vi "iRobot Navigation Target (Filtered).vi"() -> ()   [LabVIEW 2013]
uses:
  iRobot Sensors.ctl
  iRobot/Sensor/Charging State.ctl
  Accel Filtered.ctl
  iRobot Navigation State Machine.lvsc/StatechartState.ctl
  iRobot Navigation State Machine.lvsc/State.ctl
  iRobot Navigation State Machine.lvsc/Inputs.ctl
  Accelerometer.ctl
  iRobot/Sensor/Sensor Group 6.ctl
  iRobot/Sensor/Bumps + Wheel Drops.ctl
  iRobot/Sensor/Low-Side Driver + Wheel Overcurrent.ctl
  iRobot/Sensor/Buttons.ctl
  iRobot/Sensor/Cargo Bay Digital Inputs.ctl
  iRobot/Sensor/Charging Sources Available.ctl
  iRobot/Sensor/OI Mode.ctl
  <vilib>/Statechart/Common/IntGuid.ctl
  <vilib>/Statechart/Common/DbgID.ctl
  <vilib>/myRIO/Common/Instrument Driver Framework/myRIO v1.0/UART/vis/myRIO v1.0 Close UART.vi
  <vilib>/myRIO/Common/Instrument Driver Framework/myRIO v1.0/myRIO v1.1 Open.vi
  iRobot Navigation State Machine.lvsc/CompanionDiagram.vi
  iRobot Navigation State Machine.lvsc/CompanionDiagram.vi/38/SC Main.vi
  <vilib>/myRIO/Common/Instrument Driver Framework/Utilities/vis/FPGA Ref Manager.vi
  <vilib>/myRIO/Common/Instrument Driver Framework/myRIO v1.0/myRIO v1.0 Reset FPGA.vi
  iRobot Navigation State Machine.lvsc/Trigger.ctl
  <vilib>/Statechart/Infrastructure/RTStatechart/RunTime SCN.xnode
  iRobot Navigation State Machine.lvsc/Outputs.ctl
  iRobot Navigation State Machine.lvsc
  <vilib>/myRIO/Instrument Drivers/Utilities/Utilities.lvlib
  <vilib>/Statechart/Common/NI_SC_LVSCCommonFiles.lvlib
panel:
  in  "Reset Peak Deg":bool
  out "Horiz. Peak Angle 2":dbl
  in  "Delta Mag. Thresh. 2":dbl
  in  "Deg. Accel. Thresh.":dbl
  out "Horiz. Peak Angle":dbl
  in  "Reset Accel Max":bool
  in  "Reset Delta Max":bool
  in  "Tab Control":T1(tab)
  out "iRobot Sensors (graphical)":T2 {"Filtered Delta Max"."All Mag" format="%_3f"; "Filtered Delta Max"."Vert Mag" format="%_3f"; "Filtered Delta Max"."x axis (g)" format="%_3f"; "Filtered Delta Max"."y axis (g)" format="%_3f"; "Filtered Delta Max"."z axis (g)" format="%_3f"; "Filtered Delta Max"."Horiz Mag" format="%_3f"; "Filtered Accel Max"."All Mag" format="%_3f"; "Filtered Accel Max"."Vert Mag" format="%_3f"; "Filtered Accel Max"."x axis (g)" format="%_3f"; "Filtered Accel Max"."y axis (g)" format="%_3f"; "Filtered Accel Max"."z axis (g)" format="%_3f"; "Filtered Accel Max"."Horiz Mag" format="%_3f"; "Right Wheel (mm/s)" scale=-500.0..500.0; "Left Wheel (mm/s)" scale=-500.0..500.0}
  in  "Full Mode":bool
  out "Active States":T6
  out "error out":errorcluster
  in  "Wheel Speed (mm/s)":i16(slide)=100 scale=0.0..500.0
  in  "accel smoothing (0-1)":dbl=1.0
  in  "accel HPF (0-1)":dbl=0.7
  in  "stop":bool
  out "Target Running":bool
  # "Battery"
  # "Set to 1 to disable"
  # "Set to 0 to disable ???"
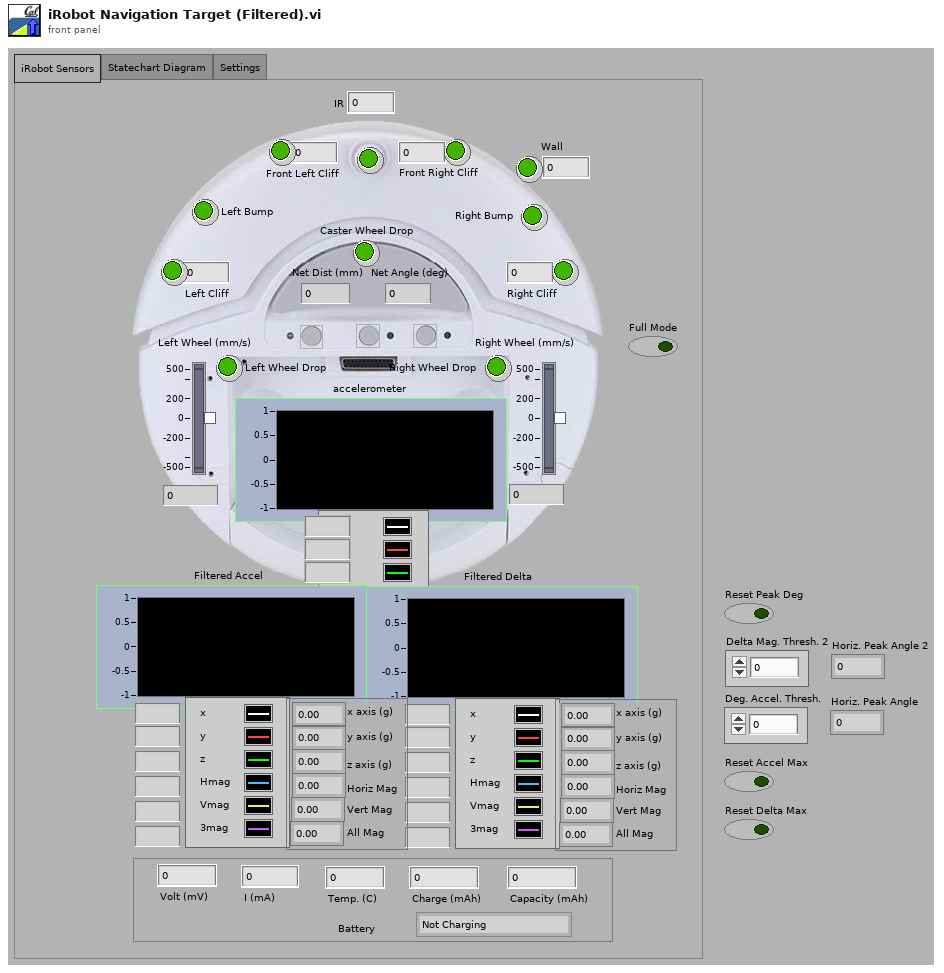
[diagram p1: front panel]
types:
  T1 = enum32{"iRobot Sensors", "Statechart Diagram", "Settings"}
  T2 = typedef "iRobot Sensors.ctl" = cluster{"Caster Wheel Drop":bool, "Left Wheel Drop":bool, "Right Wheel Drop":bool, "Left Bump":bool, "Right Bump":bool, "Left Cliff":bool, "Front Left Cliff":bool, "Front Right Cliff":bool, "Right Cliff":bool, "Wall":bool, "Net Dist (mm)":i32, "Net Angle (deg)":i32, "Wall":u16, "Left Cliff":u16, "Front Left Cliff":u16, "Front Right Cliff":u16, "Right Cliff":u16, "Left Wheel (mm/s)":i16, "Right Wheel (mm/s)":i16, "accelerometer":T3, "Virtual Wall":bool, "Volt (mV)":u16, "I (mA)":i16, "Temp. (C)":i8, "Charge (mAh)":u16, "Capacity (mAh)":u16, "Charging State":T4, "IR":u8, "Filtered Accel":cluster{"x axis (g)":dbl, "y axis (g)":dbl, "z axis (g)":dbl, "Horiz Mag":dbl, "Vert Mag":dbl, "All Mag":dbl}, "Filtered Delta":cluster{"x axis (g)":dbl, "y axis (g)":dbl, "z axis (g)":dbl, "Horiz Mag":dbl, "Vert Mag":dbl, "All Mag":dbl}, "Filtered Accel Max":T5, "Filtered Delta Max":T5}
  T3 = typedef "Accelerometer.ctl" = cluster{"x axis (g)":dbl, "y axis (g)":dbl, "z axis (g)":dbl}
  T4 = typedef "Charging State.ctl" = enum16{"Not Charging", "Reconditioning Charging", "Full Charging", "Trickle Charging", "Waiting", "Charging Fault Condition"}
  T5 = typedef "Accel Filtered.ctl" = cluster{"x axis (g)":dbl, "y axis (g)":dbl, "z axis (g)":dbl, "Horiz Mag":dbl, "Vert Mag":dbl, "All Mag":dbl}
  T6 = typedef "iRobot Navigation State Machine.lvsc/StatechartState.ctl" = T7[]
  T7 = typedef "iRobot Navigation State Machine.lvsc/State.ctl" = enum16{"NI.SC.Initial", "NI.SC.History", "NI.SC.ShallowHistory", "NI.SC.Terminal", "Pause", "Run", "Pause\\Detect Play Button\\Pause;\nWait for\nbutton\nrelease", "Pause\\Detect Play Button\\Unpause;\nwait for\nbutton release", "Pause\\Detect Play Button\\Unpause;\nwait for\nbutton press", "Run\\Detect Obstacles\\Return Right", "Run\\Detect Obstacles\\Return Left", "Run\\Detect Obstacles\\Move Forward", "Run\\Detect Obstacles\\Turn Right", "Run\\Detect Obstacles\\Turn Left", "Run\\Detect Obstacles\\Backup", "Run\\Detect Obstacles\\Drive"}
  T8 = typedef "iRobot UART Port Type.ctl" = refnum<visa-resource-name>
  T9 = typedef "NI_SC_LVSCCommonFiles.lvlib/IntGuid.ctl" = cluster{"Data1":u32, "Data2":u16, "Data3":u16, "Data4":u8, "Data5":u8, "Data6":u8, "Data11":u8, "Data9":u8, "Data10":u8, "Data8":u8, "Data7":u8}
  T10 = typedef "NI_SC_LVSCCommonFiles.lvlib/DbgID.ctl" = cluster{"VIRef":u32, "IntGUID":T9}
  T11 = typedef "iRobot Navigation State Machine.lvsc/Inputs.ctl" = cluster{"net distance (mm)":i32, "net angle (deg)":i32, "Max Wheel Speed (mm/s)":i16, "accelerometer":T3, "iRobot Sensors":T12, "Is Simulator?":bool, "Filtered Accelerometer":T5, "Filtered Accel Delta":T5}
  T12 = typedef "Sensor Group 6.ctl" = cluster{"Bumps + Wheel Drops":T13, "Wall":bool, "Cliff Left":bool, "Cliff Front Left":bool, "Cliff Front Right":bool, "Cliff Right":bool, "Virtual Wall":bool, "Low-Side Driver + Wheel Overcurrent":T14, "Infrared":u8, "Buttons":T15, "Distance (mm)":i32, "Angle (deg)":i32, "Charging State":T4, "Voltage (mV)":u16, "Current (mA)":i16, "Battery Temperature (deg C)":i8, "Battery Charge (mAh)":u16, "Battery Capacity (mAh)":u16, "Wall Signal (0-4095)":u16, "Cliff Left Signal (0-4095)":u16, "Cliff Front Left Signal (0-4095)":u16, "Cliff Front Right Signal (0-4095)":u16, "Cliff Right Signal (0-4095)":u16, "Cargo Bay Digital Inputs":T16, "Cargo Bay Analog Signal (0-1023)":u16, "Charging Sources Available":T17, "OI Mode":T18, "Song Number":u8, "Song Playing":bool, "Number of Stream Packets":u8, "Requested Velocity (mm/s)":i16, "Requested Radius (mm)":i16, "Requested Right Wheel Velocity (mm/s)":i16, "Requested Left Wheel Velocity (mm/s)":i16}
  T13 = typedef "Bumps + Wheel Drops.ctl" = cluster{"Wheeldrop Caster":bool, "Wheeldrop Left":bool, "Wheeldrop Right":bool, "Bump Left":bool, "Bump Right":bool}
  T14 = typedef "Low-Side Driver + Wheel Overcurrent.ctl" = cluster{"Low-Side Driver 0":bool, "Low-Side Driver 1":bool, "Low-Side Driver 2":bool, "Left Wheel":bool, "Right Wheel":bool}
  T15 = typedef "Buttons.ctl" = cluster{"Advance":bool, "Play":bool}
  T16 = typedef "Cargo Bay Digital Inputs.ctl" = cluster{"Digital Input 0":bool, "Digital Input 1":bool, "Digital Input 2":bool, "Digital Input 3":bool, "Device Detect":bool}
  T17 = typedef "Charging Sources Available.ctl" = cluster{"Internal Charger":bool, "Home Base":bool}
  T18 = typedef "OI Mode.ctl" = enum16{"Off", "Passive", "Safe", "Full"}
  T19 = typedef "iRobot Navigation State Machine.lvsc/Outputs.ctl" = cluster{"Left Wheel Speed (mm/s)":i16, "Right Wheel Speed (mm/s)":i16}
  T20 = cluster{"[0]":dbl, "[1]":dbl, "[2]":dbl, "[3]":dbl, "[4]":dbl, "[5]":dbl}
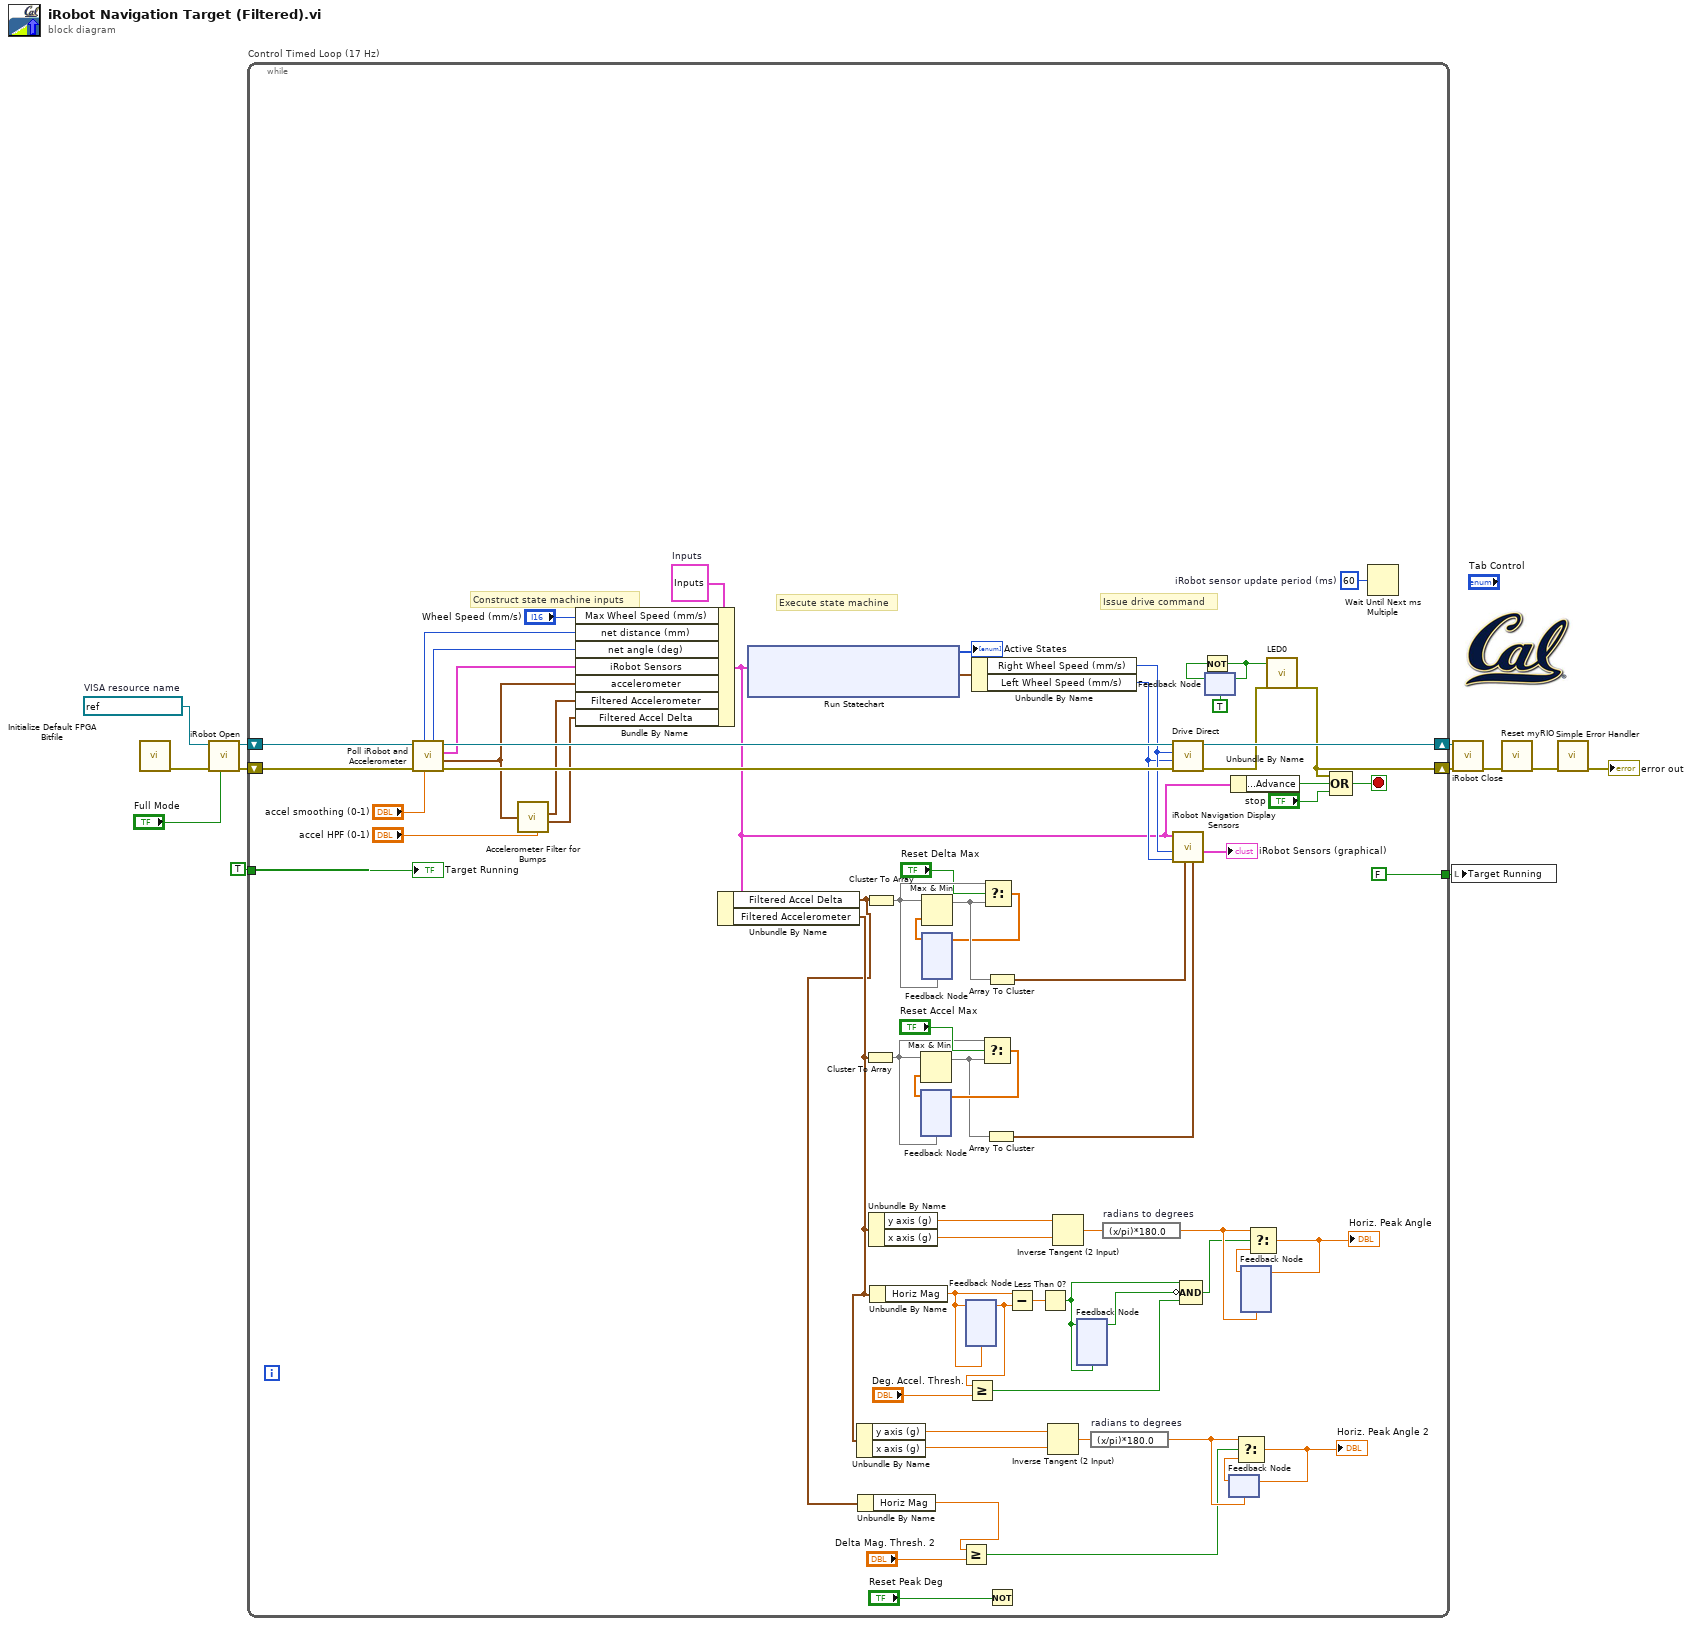
[diagram p0: block diagram]
diagram:
  w6 = refnum<visa-resource-name> "ASRL1::INSTR"  # VISA resource name
  n1 = call <vilib>:"Initialize Default FPGA Bitfile.vi"() -> ("error out"=w4:errorcluster)  [unwired: 11 in]
  n2 = call "iRobot Open.vi"("Full Mode"="Full Mode", "error in (no error)"=w4, "UART port in"=w6) -> ("error out"=w11:errorcluster, "UART port out"=w10:T8)  [unwired: 7 in]
  n3 = while "Control Timed Loop (17 Hz)" {
    shift-right: [w82] -> w12
    shift-left: w10 -> [w77]
    shift-right: [w64] -> w7
    shift-left: w11 -> [w76]
    tunnel: TRUE ("stop") -> [w70]
    tunnel: [FALSE ("stop")] -> w8
    stop <- w81 stop-if-true
    w57 = u32 60  # iRobot sensor update period (ms)
    w79 = T11 {"net distance (mm)"=0, "net angle (deg)"=0, "Max Wheel Speed (mm/s)"=0, "accelerometer"={"x axis (g)"=0.0, "y axis (g)"=0.0, "z axis (g)"=0.0}, "iRobot Sensors"={"Bumps + Wheel Drops"={"Wheeldrop Caster"=FALSE, "Wheeldrop Left"=FALSE, "Wheeldrop Right"=FALSE, "Bump Left"=FALSE, "Bump Right"=FALSE}, "Wall"=FALSE, "Cliff Left"=FALSE, "Cliff Front Left"=FALSE, "Cliff Front Right"=FALSE, "Cliff Right"=FALSE, "Virtual Wall"=FALSE, "Low-Side Driver + Wheel Overcurrent"={"Low-Side Driver 0"=FALSE, "Low-Side Driver 1"=FALSE, "Low-Side Driver 2"=FALSE, "Left Wheel"=FALSE, "Right Wheel"=FALSE}, "Infrared"=0, "Buttons"={"Advance"=FALSE, "Play"=FALSE}, "Distance (mm)"=0, "Angle (deg)"=0, "Charging State"=enum."Not Charging", "Voltage (mV)"=0, "Current (mA)"=0, "Battery Temperature (deg C)"=0, "Battery Charge (mAh)"=0, "Battery Capacity (mAh)"=0, "Wall Signal (0-4095)"=0, "Cliff Left Signal (0-4095)"=0, "Cliff Front Left Signal (0-4095)"=0, "Cliff Front Right Signal (0-4095)"=0, "Cliff Right Signal (0-4095)"=0, "Cargo Bay Digital Inputs"={"Digital Input 0"=FALSE, "Digital Input 1"=FALSE, "Digital Input 2"=FALSE, "Digital Input 3"=FALSE, "Device Detect"=FALSE}, "Cargo Bay Analog Signal (0-1023)"=0, "Charging Sources Available"={"Internal Charger"=FALSE, "Home Base"=FALSE}, "OI Mode"=enum."Off", "Song Number"=0, "Song Playing"=FALSE, "Number of Stream Packets"=0, "Requested Velocity (mm/s)"=0, "Requested Radius (mm)"=0, "Requested Right Wheel Velocity (mm/s)"=0, "Requested Left Wheel Velocity (mm/s)"=0}, "Is Simulator?"=FALSE, "Filtered Accelerometer"={"x axis (g)"=0.0, "y axis (g)"=0.0, "z axis (g)"=0.0, "Horiz Mag"=0.0, "Vert Mag"=0.0, "All Mag"=0.0}, "Filtered Accel Delta"={"x axis (g)"=0.0, "y axis (g)"=0.0, "z axis (g)"=0.0, "Horiz Mag"=0.0, "Vert Mag"=0.0, "All Mag"=0.0}}  # Inputs
    # "Issue drive command"
    # "Execute state machine"
    # "Construct state machine inputs"
    n4 = call "Poll iRobot and Accelerometer.vi"("accel smoothing (0-1)"="accel smoothing (0-1)", "error in"=w76, "UART port in"=w77) -> ("error out"=w75:errorcluster, "Acceleration (g)"=w54:T3, "iRobot SensorGroup6"=w63:T12, "UART port out"=w74:T8, "net angle (deg)"=w72:i32, "net distance (mm)"=w73:i32)  [unwired: 3 in]
    n5 = call "Accelerometer Filter for Bumps.vi"("filter factor (0-1)"="accel HPF (0-1)", "accelerometer (g)"=w54) -> ("filtered out"=w53:T5, "abs delta"=w52:T5)  [unwired: 4 in]
    n6 = Bundle By Name(cluster=w79, "Max Wheel Speed (mm/s)"="Wheel Speed (mm/s)", "net distance (mm)"=w73, "net angle (deg)"=w72, "iRobot Sensors"=w63, "accelerometer"=w54, "Filtered Accelerometer"=w53, "Filtered Accel Delta"=w52) -> (w47:T11)
    n7 = Unbundle By Name(w47) -> ("Filtered Accel Delta"=w22:T5, "Filtered Accelerometer"=w23:T5)
    n8 = xnode "Run Statechart"("Inputs"=w47) -> ("Outputs"=w80:T19, "Active States"=→"Active States":T6)  [unwired: 2 in, 1 out]
    n9 = Unbundle By Name(w23) -> ("y axis (g)"=w20:dbl, "x axis (g)"=w19:dbl)
    n10 = Unbundle By Name(w22) -> ("Horiz Mag"=w21:dbl)
    n11 = Cluster To Array(cluster=w23) -> (array=w42:dbl[])
    n12 = Cluster To Array(cluster=w22) -> (array=w49:dbl[])
    n13 = Unbundle By Name(w23) -> ("y axis (g)"=w16:dbl, "x axis (g)"=w15:dbl)
    n14 = Unbundle By Name(w23) -> ("Horiz Mag"=w30:dbl)
    n15 = feedback #1(w42) -> (w43:dbl[])
    n16 = Max & Min(x=w42, y=w43) -> (max(x,y)=w40:dbl[])  [unwired: 1 out]
    n17 = feedback #2(w49) -> (w48:dbl[])
    n18 = Max & Min(x=w49, y=w48) -> (max(x,y)=w51:dbl[])  [unwired: 1 out]
    n19 = Greater Or Equal?(x=w21, y="Delta Mag. Thresh. 2") -> (x >= y?=w13:bool)
    n20 = feedback #3(w30) -> (w28:dbl)
    n21 = feedback-in #3(w30) -> ()
    n22 = Greater Or Equal?(x=w28, y="Deg. Accel. Thresh.") -> (x >= y?=w31:bool)
    n23 = Unbundle By Name(w80) -> ("Right Wheel Speed (mm/s)"=w61:i16, "Left Wheel Speed (mm/s)"=w60:i16)
    n24 = Select(t=w42, s="Reset Accel Max", f=w40) -> (s? t:f=w41:dbl[])
    n25 = feedback-in #1(w41) -> ()
    n26 = Select(t=w49, s="Reset Delta Max", f=w51) -> (s? t:f=w50:dbl[])
    n27 = feedback-in #2(w50) -> ()
    n28 = Array To Cluster(array=w40) -> (cluster=w39:T20)
    n29 = Array To Cluster(array=w51) -> (cluster=w46:T20)
    n30 = Not(x="Reset Peak Deg") -> ()  [unwired: 1 out]
    n31 = Subtract(x=w30, y=w28) -> (x-y=w35:dbl)
    n32 = Less Than 0?(x=w35) -> (x < 0?=w29:bool)
    n33 = Inverse Tangent (2 Input)(1:w19, 2:w20) -> (0:w18:dbl)
    n34 = Inverse Tangent (2 Input)(1:w15, 2:w16) -> (0:w17:dbl)
    n35 = feedback #4(w29) -> (w34:bool)
    n36 = feedback-in #4(w29) -> ()
    n37 = expression code="(x/pi)*180.0" "radians to degrees"(w18) -> (w26:dbl)
    n38 = expression code="(x/pi)*180.0" "radians to degrees"(w17) -> (w36:dbl)
    n39 = call "Drive Direct.vi"("error in"=w75, "Left Wheel Velocity (mm/s)"=w60, "Right Wheel Velocity (mm/s)"=w61, "UART port in"=w74) -> ("error out"=w65:errorcluster, "UART port out"=w82:T8)  [unwired: 6 in]
    n40 = call "iRobot Navigation Display Sensors.vi"("Filtered Accel Max"=w39, "Filtered Delta Max"=w46, "Left Wheel (mm/s)"=w60, "Right Wheel (mm/s)"=w61, "Statechart Inputs"=w47) -> ("iRobot Sensors (graphical)"=→"iRobot Sensors (graphical)":T2)  [unwired: 4 in]
    n41 = Compound Arithmetic op=AND(w29, invert w34, w31) -> (w33:bool)
    n42 = feedback #5(TRUE) -> (w66:bool)
    n43 = Not(x=w66) -> (.not. x?=w67:bool)
    n44 = feedback-in #5(w67) -> ()
    n45 = feedback #6(w26) -> (w24:dbl)
    n46 = Unbundle By Name(w47) -> ("iRobot Sensors.Buttons.Advance"=w58:bool)
    n47 = Select(t=w26, s=w13, f=w24) -> (s? t:f=w25:dbl)
    "Horiz. Peak Angle 2" <- w25
    n48 = feedback-in #6(w25) -> ()
    n49 = feedback #7(w36) -> (w38:dbl)
    n50 = Select(t=w36, s=w33, f=w38) -> (s? t:f=w37:dbl)
    "Horiz. Peak Angle" <- w37
    n51 = feedback-in #7(w37) -> ()
    n52 = call "LED0"("LED0"=w67, "error in (no error)"=w65) -> ("error out"=w64:errorcluster)  [unwired: 25 in]
    n53 = Compound Arithmetic op=OR(w64, w58, "stop") -> (w81:bool)
    n54 = Wait Until Next ms Multiple(millisecond multiple=w57) -> ()  [unwired: 1 out]
    "Target Running" <- w70
  }
  n55 = local write "Target Running"(w8) -> ()
  n56 = call "iRobot Close.vi"("error in"=w7, "UART port in"=w12) -> ("error out"=w2:errorcluster)  [unwired: 9 in]
  n57 = call <vilib>:"Reset myRIO.vi"("error in (no error)"=w2) -> ("error out"=w5:errorcluster)  [unwired: 10 in]
  n58 = call <vilib>:"Simple Error Handler.vi"("error in (no error)"=w5) -> ("error out"=→"error out":errorcluster)  [unwired: 4 in, 4 out]
